vi "poll.vi"(8 "error in (no error)":errorcluster, 11 "output_actor in":refnum<class "Output Actor.lvclass">) -> (0 "error out":errorcluster)   [LabVIEW 2015, in "Output Actor.lvclass"]
uses:
  Output Actor.lvclass
  <vilib>/ActorFramework/Actor/Actor.lvclass/Actor.ctl
  <vilib>/ActorFramework/Message Enqueuer/Message Enqueuer.lvclass/Message Enqueuer.ctl
  <vilib>/ActorFramework/Message Enqueuer/Enqueue.vi
  <vilib>/ActorFramework/Message Enqueuer/Init from Existing Queue.vi
  <vilib>/ActorFramework/Message Priority Queue/Priority Enqueue.vi
  <vilib>/ActorFramework/Stop Msg/Stop Msg.lvclass
  <vilib>/ActorFramework/Message Enqueuer/Message Enqueuer.lvclass
  <vilib>/ActorFramework/Actor/Actor.lvclass
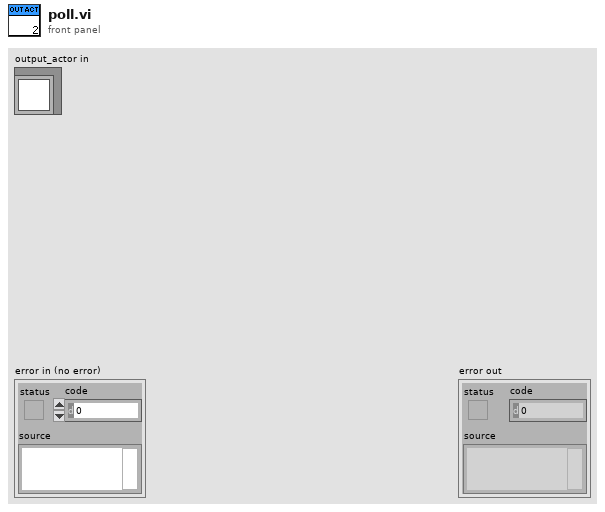
[diagram p1: front panel]
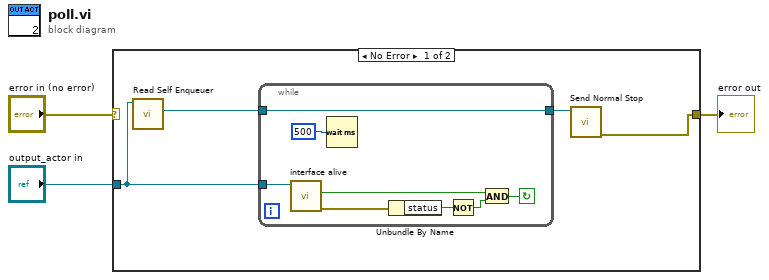
[diagram p0: block diagram]
diagram:
  n1 = case shown="No Error" "error in (no error)" {
    selector: "error in (no error)" -> [_ w16]
    tunnel: [w6 w16] -> w2
    tunnel: "output_actor in" -> [w7 _]
    frame No Error {
      n2 = call <vilib>:"Read Self Enqueuer.vi"("Actor"=w7) -> ("Self Enqueuer"=w4:refnum<class "Message Enqueuer.lvclass">)  [unwired: 10 in]
      n3 = while {
        tunnel: w7 -> [w15]
        tunnel: [w8] -> w5
        tunnel: w4 -> [w8]
        stop <- w10 continue-if-true
        n4 = call "interface alive.vi"("output_actor in"=w15) -> ("error out"=w14:errorcluster, "alive"=w11:bool)  [unwired: 8 in, 1 out]
        n5 = Wait (ms)(milliseconds to wait=u32 500) -> ()  [unwired: 1 out]
        n6 = Unbundle By Name(w14) -> ("status"=w13:bool)
        n7 = Not(x=w13) -> (.not. x?=w12:bool)
        n8 = And(x=w11, y=w12) -> (x .and. y?=w10:bool)
      }
      n9 = call <vilib>:"Send Normal Stop.vi"("Message Enqueuer"=w5) -> ("error out"=w6:errorcluster)  [unwired: 10 in]
    }
    frame Error {
    }
  }
  "error out" <- w2
